vi "Calibrate.vi"(6 "Calibrate Axis":enum8{"Z", "X", "Y"}(ring), 7 "Port":T1 items=["Port 1", "Port 2", "Port 3", "Port 4"], 9 "Accel Input Array":dbl[](array[numeric])=[0.0, 0.0, 0.0], 11 "NXT":T2) -> (3 "NXT":T2)   [LabVIEW 2010]
uses:
  <vilib>/NXT/Subs/LVHSConnector.ctl
  <vilib>/NXT/Block Support/NXT_InputPort.ctl
  <vilib>/NXT/Dual Mode Library/prims/dataManipulation/splitU16.vi
  <vilib>/NXT/Dual Mode Library/Sensors/i2c_sensors.vi
panel:
  # "Z = 0\nX = 1\nY = 2"
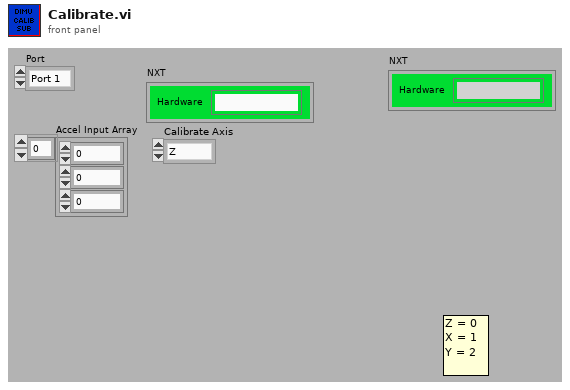
[diagram p1: front panel]
types:
  T1 = typedef "NXT_InputPort.ctl" = u8
  T2 = typedef "LVHSConnector.ctl" = cluster{"Hardware":string, "Flattened String":string}
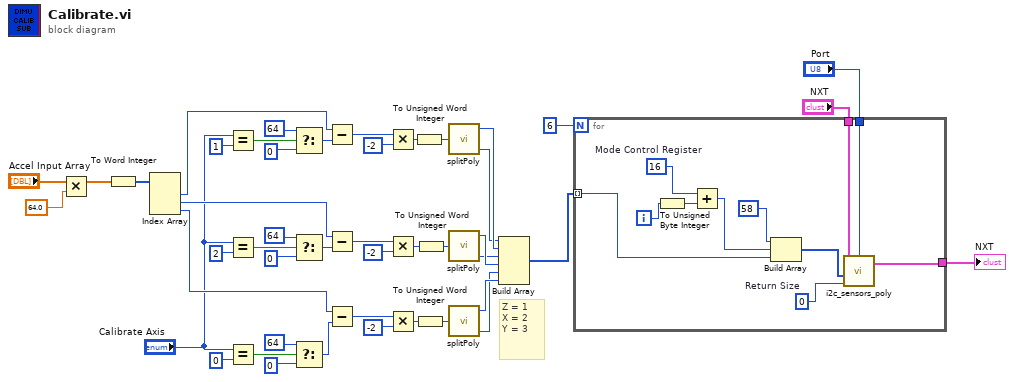
[diagram p0: block diagram]
diagram:
  # "Z = 1\nX = 2\nY = 3"
  n1 = Multiply(x="Accel Input Array", y=64.0) -> (x*y=w11:dbl[])
  n2 = To Word Integer(number=w11) -> (16bit integer=w6:i16[])
  n3 = Index Array(array=w6) -> (element #1=w5:i16, element #2=w4:i16, element #3=w3:i16)  [unwired: 3 in]
  n4 = Equal?(x="Calibrate Axis", y=u8 1) -> (x = y?=w18:bool)
  n5 = Equal?(x="Calibrate Axis", y=u8 2) -> (x = y?=w24:bool)
  n6 = Equal?(x="Calibrate Axis", y=u8 0) -> (x = y?=w30:bool)
  n7 = Select(t=i16 64, s=w18, f=i16 0) -> (s? t:f=w15:i16)
  n8 = Select(t=i16 64, s=w24, f=i16 0) -> (s? t:f=w20:i16)
  n9 = Select(t=i16 64, s=w30, f=i16 0) -> (s? t:f=w26:i16)
  n10 = Subtract(x=w5, y=w15) -> (x-y=w14:i16)
  n11 = Subtract(x=w4, y=w20) -> (x-y=w19:i16)
  n12 = Subtract(x=w3, y=w26) -> (x-y=w25:i16)
  n13 = Multiply(x=w14, y=i16 -2) -> (x*y=w45:i16)
  n14 = Multiply(x=w19, y=i16 -2) -> (x*y=w43:i16)
  n15 = Multiply(x=w25, y=i16 -2) -> (x*y=w32:i16)
  n16 = To Unsigned Word Integer(number=w45) -> (unsigned 16bit integer=w9:u16)
  n17 = To Unsigned Word Integer(number=w32) -> (unsigned 16bit integer=w7:u16)
  n18 = To Unsigned Word Integer(number=w43) -> (unsigned 16bit integer=w8:u16)
  n19 = call-poly <vilib>:"splitPoly.vi"("x"=w9) -> ("lo(x)"=w37:u8, "hi(x)"=w38:u8)  [unwired: 3 in]
  n20 = call-poly <vilib>:"splitPoly.vi"("x"=w8) -> ("lo(x)"=w35:u8, "hi(x)"=w36:u8)  [unwired: 3 in]
  n21 = call-poly <vilib>:"splitPoly.vi"("x"=w7) -> ("lo(x)"=w33:u8, "hi(x)"=w34:u8)  [unwired: 3 in]
  n22 = Build Array(w37, w38, w35, w36, w33, w34) -> (w31:u8[])
  n23 = for {
    N: 6 -> [_]
    tunnel: w31 -> [w54] mode=indexing
    tunnel: "Port" -> [w53]
    tunnel: "NXT" -> [w52]
    tunnel: [w51] -> w39
    i -> [w50]
    w56 = u8 0  # Return Size
    w49 = u8 16  # Mode Control Register
    n24 = To Unsigned Byte Integer(number=w50) -> (unsigned 8bit integer=w47:u8)
    n25 = Add(x=w49, y=w47) -> (x+y=w48:u8)
    n26 = Build Array(u8 58 ("element"), w48, w54) -> (w57:u8[])
    n27 = call-poly <vilib>:"i2c_sensors_poly.vi"("Return Length"=w56, "Bytes to Write"=w57, "NXT"=w52, "Port"=w53) -> ("NXT"=w51:T2)  [unwired: 1 in, 2 out]
  }
  "NXT" <- w39
